vi "z_scan_readv3.vi"(11 "address in":u32) -> (1 "intensity":i16, 2 "z-value":i16, 3 "address out":u32)   [LabVIEW 2010]
uses:
  <vilib>/rvi/DataTransferAndStorage/Container/XNode/niFpgaContainer.xnode
  <vilib>/rvi/Memory/Memory_Emulation/nirvimemoryEmulationManagerCache_GetValue.vi
  <vilib>/rvi/DataTransferAndStorage/Container/Common/niFpgaContainerGetUniqueNameForEmu.vi
  <vilib>/rvi/Memory/Memory_Emulation/nirvimemoryEmulationManagerCache_InsertValue.vi
  <vilib>/Utility/error.llb/Clear Errors.vi
  <vilib>/rvi/Memory/Memory_Emulation/nirvimemoryEmulationManagerCache_SetValue.vi
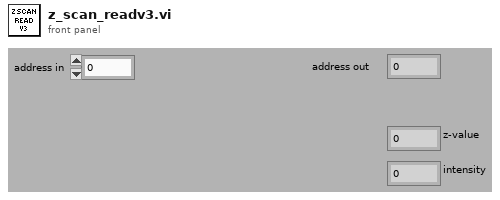
[diagram p1: front panel]
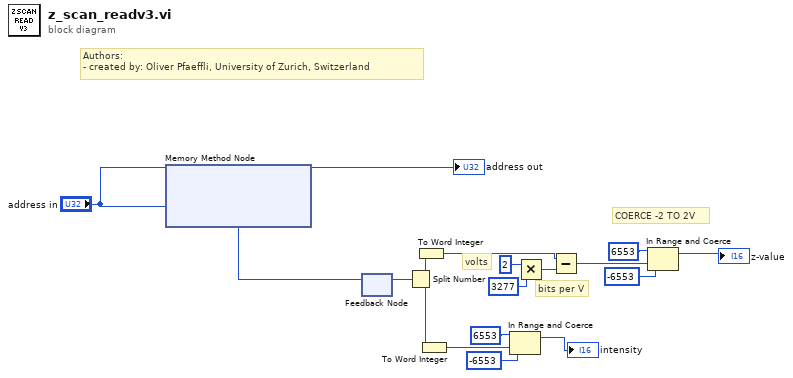
[diagram p0: block diagram]
diagram:
  # "COERCE -2 TO 2V"
  # "bits per V"
  # "volts"
  # "Authors: \n- created by: Oliver Pfaeffli, University of Zurich, Switzerland"
  n1 = xnode ("Memory Method Node")("Address"="address in") -> ("Data"=w14:u32)  [unwired: 1 in, 1 out]
  n2 = feedback #1() -> (w13:u32)  [unwired: 1 in]
  n3 = feedback-in #1(w14) -> ()
  n4 = Split Number(x=w13) -> (hi(x)=w16:u16, lo(x)=w15:u16)
  n5 = To Word Integer(number=w16) -> (16bit integer=w6:i16)
  n6 = To Word Integer(number=w15) -> (16bit integer=w2:i16)
  n7 = In Range and Coerce(upper limit=i16 6553, x=w2, lower limit=i16 -6553) -> (coerced(x)=→"intensity":i16)  [unwired: 1 out]
  n8 = Multiply(x=i16 2 ("y"), y=i16 3277) -> (x*y=w11:i16)
  n9 = Subtract(x=w6, y=w11) -> (x-y=w7:i16)
  n10 = In Range and Coerce(upper limit=i16 6553, x=w7, lower limit=i16 -6553) -> (coerced(x)=→"z-value":i16)  [unwired: 1 out]
  "address out" <- "address in"
